vi "Build Transmission Sequence.vi"(8 "error in":errorcluster, 11 "Data":variant) -> (0 "error out":errorcluster, 3 "Transmission Sequence":u8[](array[numeric]) format="%.0x")   [LabVIEW 2024, in "CANopen.lvlib" / "CANopen.lvclass"]
doc: "For transmission across the network a bit sequence is reordered into a sequence of octets."
uses:
  CANopen.lvclass
  CANopen.lvclass/CANopen.ctl
  <userlib>/_OpenG.lib/lvdata/lvdata.llb/openg_variant.lvlib
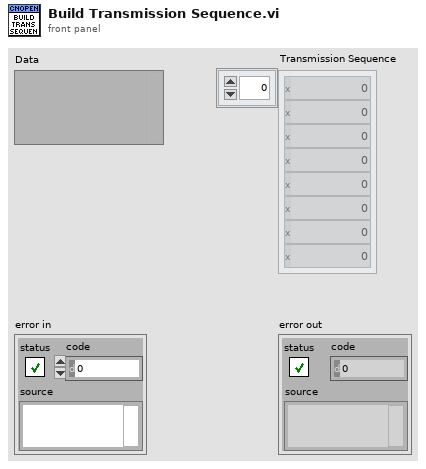
[diagram p1: front panel]
types:
  T1 = typedef "openg_variant.lvlib/Type Descriptor Enumeration__ogtk.ctl" = enum8{"<Null>", "I8", "I16", "I32", "I64", "U8", "U16", "U32", "U64", "SGL", "DBL", "EXT", "CSG", "CDB", "CXT", "0x0F", "0x10", "0x11", "0x12", "0x13", "0x14", "Enum U8", "Enum U16", "Enum U32", "Enum U64", "SGL PQ", "DBL PQ", "EXT PQ", "CSG PQ", "CDB PQ", "CXT PQ", "0x1F", "0x20", "Boolean", "0x22", "0x23", "0x24", "0x25", "0x26", "0x27", "0x28", "0x29", "0x2A", "0x2B", "0x2C", "0x2D", "0x2E", "0x2F", "String", "0x31", "Path", "Pict", "0x34", "0x35", "0x36", "DAQ", "0x38", "0x39", "0x3A", "0x3B", "0x3C", "0x3D", "0x3E", "0x3F", "Array", "0x41", "0x42", "0x43", "0x44", "0x45", "0x46", "0x47", "0x48", "0x49", "0x4A", "0x4B", "0x4C", "0x4D", "0x4E", "0x4F", "Cluster", "0x51", "0x52", "Variant", "Waveform", "0x55", "0x56", "0x57", "0x58", "0x59", "0x5A", "0x5B", "0x5C", "0x5D", "0x5E", "Fixed Point", "0x60", "0x61", "0x62", "0x63", "0x64", "0x65", "0x66", "0x67", "0x68", "0x69", "0x6A", "0x6B", "0x6C", "0x6D", "0x6E", "0x6F", "Refnum", "0x71", "0x72", "Set Collection", "Map Collection"}
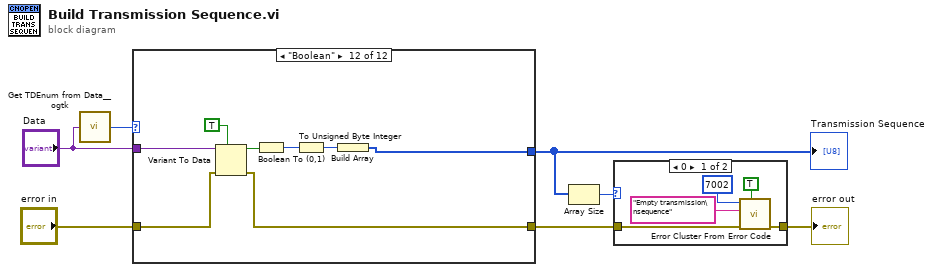
[diagram p0: block diagram]
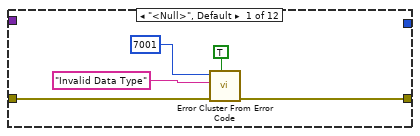
[diagram p3: hidden frame]
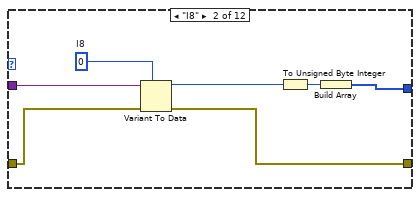
[diagram p4: hidden frame]
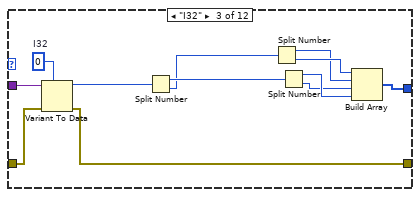
[diagram p5: hidden frame]
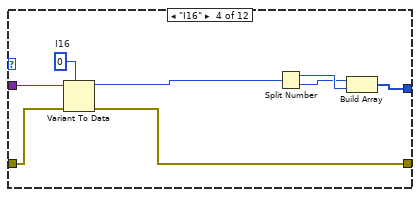
[diagram p6: hidden frame]
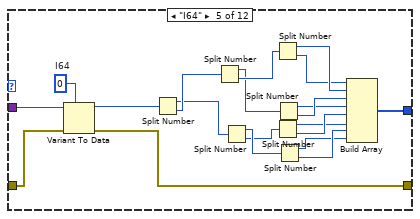
[diagram p7: hidden frame]
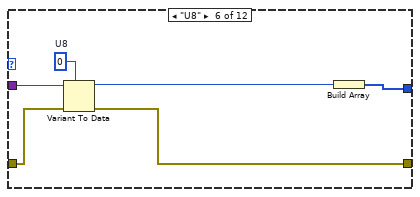
[diagram p8: hidden frame]
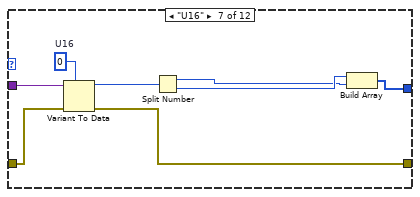
[diagram p9: hidden frame]
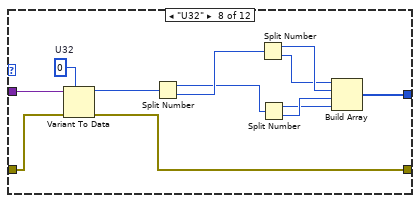
[diagram p10: hidden frame]
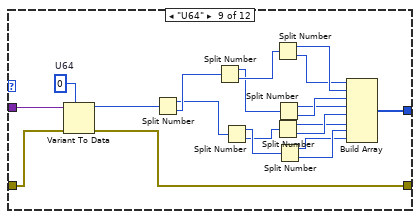
[diagram p11: hidden frame]
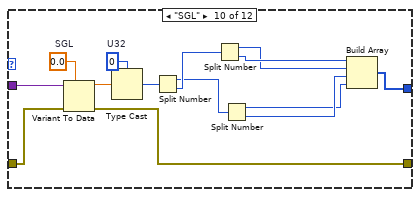
[diagram p12: hidden frame]
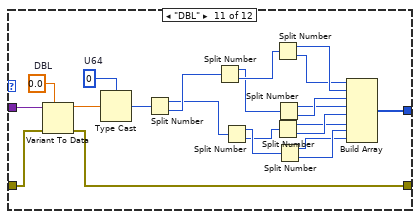
[diagram p13: hidden frame]
diagram:
  n1 = call <userlib>:"Get TDEnum from Data__ogtk.vi"("Data"="Data") -> ("Type Descriptor Enumeration"=w7:T1)  [unwired: 4 in]
  n2 = case shown="\"Boolean\"" w7 {
    tunnel: "Data" -> [_ w19 w31 w38 w58 w64 w72 w84 w104 w118 w140 w148]
    tunnel: "error in" -> [w12 w18 w30 w37 w57 w63 w71 w83 w103 w117 w139 w147]
    tunnel: [w11 w17 w29 w36 w56 w62 w70 w82 w102 w116 w138 w144] -> w4
    tunnel: [_ w14 w22 w34 w53 w61 w66 w79 w99 w110 w135 w143] -> w2
    frame "<Null>", Default {
      n3 = call <vilib>:"Error Cluster From Error Code.vi"("show call chain? (False)"=TRUE, "error in (no error)"=w12, "error message (\"\")"="Invalid Data Type" ("error message (\"\")"), "error code (0)"=7001) -> ("error out"=w11:errorcluster)  [unwired: 5 in]
    }
    frame "I8" {
      w16 = i8 0  # I8
      n4 = Variant To Data(error in=w18, type=w16, Variant=w19) -> (data=w15:i8, error out=w17:errorcluster)
      n5 = To Unsigned Byte Integer(number=w15) -> (unsigned 8bit integer=w13:u8)
      n6 = Build Array(w13) -> (w14:u8[])
    }
    frame "I32" {
      w28 = 0  # I32
      n7 = Variant To Data(error in=w30, type=w28, Variant=w31) -> (data=w23:i32, error out=w29:errorcluster)
      n8 = Split Number(x=w23) -> (hi(x)=w27:u16, lo(x)=w21:u16)
      n9 = Split Number(x=w21) -> (hi(x)=w24:u8, lo(x)=w25:u8)
      n10 = Split Number(x=w27) -> (hi(x)=w26:u8, lo(x)=w20:u8)
      n11 = Build Array(w25, w24, w20, w26) -> (w22:u8[])
    }
    frame "I16" {
      w39 = i16 0  # I16
      n12 = Variant To Data(error in=w37, type=w39, Variant=w38) -> (data=w35:i16, error out=w36:errorcluster)
      n13 = Split Number(x=w35) -> (hi(x)=w33:u8, lo(x)=w32:u8)
      n14 = Build Array(w32, w33) -> (w34:u8[])
    }
    frame "I64" {
      w59 = i64 0  # I64
      n15 = Variant To Data(error in=w57, type=w59, Variant=w58) -> (data=w55:i64, error out=w56:errorcluster)
      n16 = Split Number(x=w55) -> (hi(x)=w50:u32, lo(x)=w51:u32)
      n17 = Split Number(x=w51) -> (hi(x)=w46:u16, lo(x)=w47:u16)
      n18 = Split Number(x=w50) -> (hi(x)=w49:u16, lo(x)=w48:u16)
      n19 = Split Number(x=w47) -> (hi(x)=w54:u8, lo(x)=w52:u8)
      n20 = Split Number(x=w48) -> (hi(x)=w42:u8, lo(x)=w43:u8)
      n21 = Split Number(x=w46) -> (hi(x)=w44:u8, lo(x)=w45:u8)
      n22 = Split Number(x=w49) -> (hi(x)=w40:u8, lo(x)=w41:u8)
      n23 = Build Array(w52, w54, w45, w44, w43, w42, w41, w40) -> (w53:u8[])
    }
    frame "U8" {
      w65 = u8 0  # U8
      n24 = Variant To Data(error in=w63, type=w65, Variant=w64) -> (data=w60:u8, error out=w62:errorcluster)
      n25 = Build Array(w60) -> (w61:u8[])
    }
    frame "U16" {
      w73 = u16 0  # U16
      n26 = Variant To Data(error in=w71, type=w73, Variant=w72) -> (data=w69:u16, error out=w70:errorcluster)
      n27 = Split Number(x=w69) -> (hi(x)=w67:u8, lo(x)=w68:u8)
      n28 = Build Array(w68, w67) -> (w66:u8[])
    }
    frame "U32" {
      w85 = u32 0  # U32
      n29 = Variant To Data(error in=w83, type=w85, Variant=w84) -> (data=w81:u32, error out=w82:errorcluster)
      n30 = Split Number(x=w81) -> (hi(x)=w74:u16, lo(x)=w75:u16)
      n31 = Split Number(x=w75) -> (hi(x)=w80:u8, lo(x)=w78:u8)
      n32 = Split Number(x=w74) -> (hi(x)=w76:u8, lo(x)=w77:u8)
      n33 = Build Array(w78, w80, w77, w76) -> (w79:u8[])
    }
    frame "U64" {
      w105 = u64 0  # U64
      n34 = Variant To Data(error in=w103, type=w105, Variant=w104) -> (data=w101:u64, error out=w102:errorcluster)
      n35 = Split Number(x=w101) -> (hi(x)=w96:u32, lo(x)=w97:u32)
      n36 = Split Number(x=w97) -> (hi(x)=w92:u16, lo(x)=w93:u16)
      n37 = Split Number(x=w96) -> (hi(x)=w95:u16, lo(x)=w94:u16)
      n38 = Split Number(x=w93) -> (hi(x)=w100:u8, lo(x)=w98:u8)
      n39 = Split Number(x=w94) -> (hi(x)=w88:u8, lo(x)=w89:u8)
      n40 = Split Number(x=w92) -> (hi(x)=w90:u8, lo(x)=w91:u8)
      n41 = Split Number(x=w95) -> (hi(x)=w86:u8, lo(x)=w87:u8)
      n42 = Build Array(w98, w100, w91, w90, w89, w88, w87, w86) -> (w99:u8[])
    }
    frame "SGL" {
      w111 = u32 0  # U32
      w119 = sgl 0.0  # SGL
      n43 = Variant To Data(error in=w117, type=w119, Variant=w118) -> (data=w115:sgl, error out=w116:errorcluster)
      n44 = Type Cast(type=w111, x=w115) -> (*(type *) &x=w112:u32)
      n45 = Split Number(x=w112) -> (hi(x)=w113:u16, lo(x)=w114:u16)
      n46 = Split Number(x=w114) -> (hi(x)=w108:u8, lo(x)=w109:u8)
      n47 = Split Number(x=w113) -> (hi(x)=w106:u8, lo(x)=w107:u8)
      n48 = Build Array(w109, w108, w107, w106) -> (w110:u8[])
    }
    frame "DBL" {
      w120 = u64 0  # U64
      w141 = 0.0  # DBL
      n49 = Variant To Data(error in=w139, type=w141, Variant=w140) -> (data=w137:dbl, error out=w138:errorcluster)
      n50 = Type Cast(type=w120, x=w137) -> (*(type *) &x=w121:u64)
      n51 = Split Number(x=w121) -> (hi(x)=w132:u32, lo(x)=w133:u32)
      n52 = Split Number(x=w133) -> (hi(x)=w128:u16, lo(x)=w129:u16)
      n53 = Split Number(x=w132) -> (hi(x)=w131:u16, lo(x)=w130:u16)
      n54 = Split Number(x=w129) -> (hi(x)=w136:u8, lo(x)=w134:u8)
      n55 = Split Number(x=w130) -> (hi(x)=w124:u8, lo(x)=w125:u8)
      n56 = Split Number(x=w128) -> (hi(x)=w126:u8, lo(x)=w127:u8)
      n57 = Split Number(x=w131) -> (hi(x)=w122:u8, lo(x)=w123:u8)
      n58 = Build Array(w134, w136, w127, w126, w125, w124, w123, w122) -> (w135:u8[])
    }
    frame "Boolean" {
      n59 = Variant To Data(error in=w147, type=TRUE, Variant=w148) -> (data=w146:bool, error out=w144:errorcluster)
      n60 = Boolean To (0,1)(Boolean=w146) -> (0, 1=w145:i16)
      n61 = To Unsigned Byte Integer(number=w145) -> (unsigned 8bit integer=w142:u8)
      n62 = Build Array(w142) -> (w143:u8[])
    }
  }
  "Transmission Sequence" <- w2
  n63 = Array Size(array=w2) -> (size(s)=w1:i32)
  n64 = case shown="0" w1 {
    tunnel: w4 -> [w154 w155]
    tunnel: [w153 w155] -> w3
    frame 0 {
      n65 = call <vilib>:"Error Cluster From Error Code.vi"("show call chain? (False)"=TRUE, "error in (no error)"=w154, "error message (\"\")"="Empty transmission\nsequence" ("error message (\"\")"), "error code (0)"=7002) -> ("error out"=w153:errorcluster)  [unwired: 5 in]
    }
    frame Default {
    }
  }
  "error out" <- w3
